vi "Magnet Read Message.vi"(8 "error in (no error)":errorcluster, 11 "Queue in":refnum<queue>) -> (0 "error out":errorcluster, 1 "Message Data":variant, 2 "String":string, 3 "Queue out":refnum<queue>)   [LabVIEW 2017, in "Magnet module.lvlib"]
uses:
  Magnet module.lvlib
  ctl/MSG to magnet.ctl
  ctl/Magnet Orders.ctl
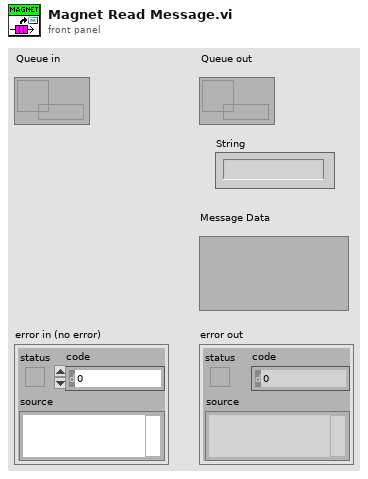
[diagram p1: front panel]
types:
  T1 = typedef "Magnet module.lvlib/MSG to magnet.ctl" = cluster{"Order":T2, "Data":variant}
  T2 = typedef "Magnet module.lvlib/Magnet Orders.ctl" = enum16{"Ignore", "Initialize", "Update", "Switch mode", "Set field", "Stop ramping", "Equalize output", "Zero output", "Blackout", "End"}
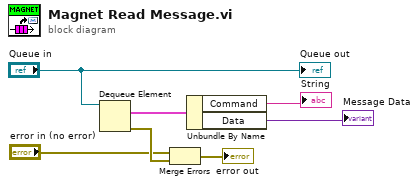
[diagram p0: block diagram]
diagram:
  n1 = Dequeue Element(queue="Queue in") -> (element=w5:T1, error out=w4:errorcluster)  [unwired: 2 in, 2 out]
  n2 = Merge Errors("error in (no error)", w4) -> (→"error out":errorcluster)
  n3 = Unbundle By Name(w5) -> ("Command"=→"String":string, "Data"=→"Message Data":variant)
  "Queue out" <- "Queue in"
